vi "Get Min Max.vi"(10 "Axis":T1, 11 "Hailstone in":refnum<class "Hailstone.lvclass">) -> (3 "Limits":cluster{"Min":i64, "Max":i64})   [LabVIEW 2021, in "Hailstone.lvclass"]
uses:
  Hailstone.lvclass
  Axis.ctl
  Hailstone.lvclass/Hailstone.ctl
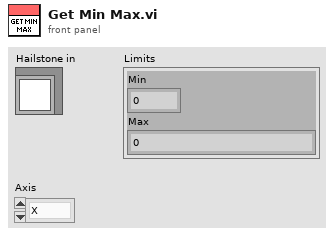
[diagram p1: front panel]
types:
  T1 = typedef "Hailstone.lvclass/Axis.ctl" = enum16{"X", "Y", "Z"}
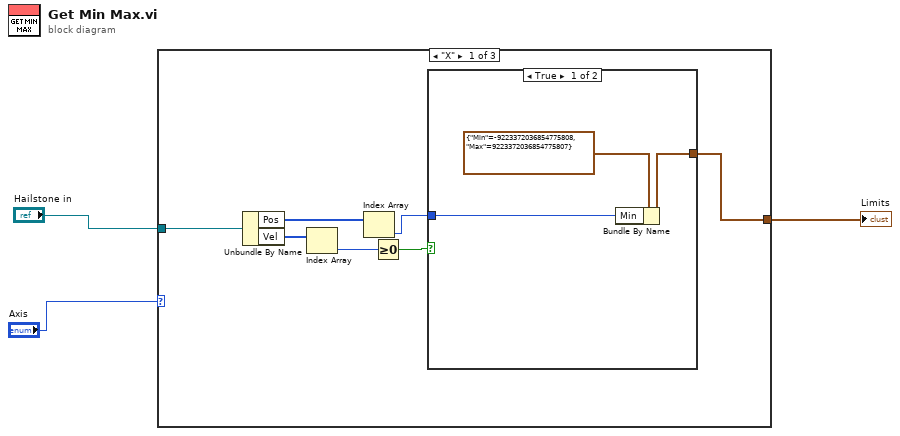
[diagram p0: block diagram]
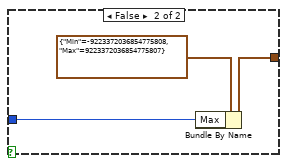
[diagram p2: hidden frame]
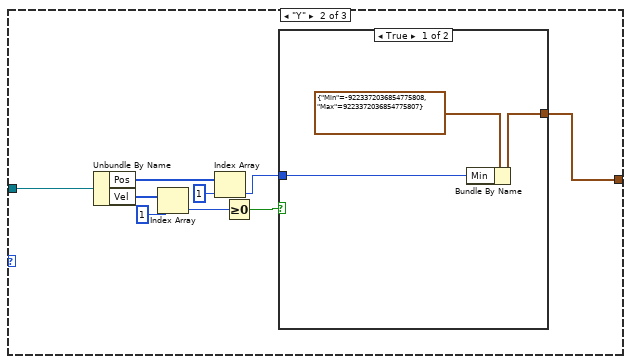
[diagram p3: hidden frame]
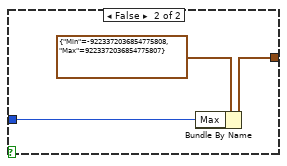
[diagram p4: hidden frame]
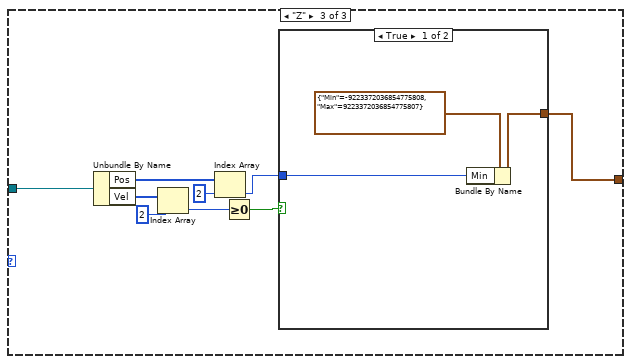
[diagram p5: hidden frame]
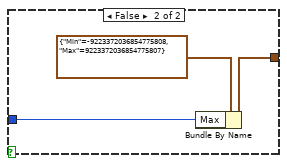
[diagram p6: hidden frame]
diagram:
  n1 = case shown="\"X\"" "Axis" {
    tunnel: "Hailstone in" -> [w10 w25 w40]
    tunnel: [w6 w21 w36] -> w2
    frame "X" {
      n2 = Unbundle By Name(w10) -> ("Pos"=w5:i64[], "Vel"=w9:i64[])
      n3 = Index Array(array=w9) -> (element=w8:i64)  [unwired: 1 in]
      n4 = Index Array(array=w5) -> (element=w4:i64)  [unwired: 1 in]
      n5 = Greater Or Equal To 0?(x=w8) -> (x >= 0?=w7:bool)
      n6 = case shown="True" w7 {
        tunnel: [w12 w15] -> w6
        tunnel: w4 -> [w11 w14]
        frame True {
          n7 = Bundle By Name(cluster=cluster{"Min":i64, "Max":i64} {"Min"=-9223372036854775808, "Max"=9223372036854775807} ("Limits"), "Min"=w11) -> (w12:cluster{"Min":i64, "Max":i64})
        }
        frame False {
          n8 = Bundle By Name(cluster=cluster{"Min":i64, "Max":i64} {"Min"=-9223372036854775808, "Max"=9223372036854775807} ("Limits"), "Max"=w14) -> (w15:cluster{"Min":i64, "Max":i64})
        }
      }
    }
    frame "Y" {
      n9 = Unbundle By Name(w25) -> ("Pos"=w20:i64[], "Vel"=w24:i64[])
      n10 = Index Array(array=w24, index=1) -> (element=w23:i64)
      n11 = Index Array(array=w20, index=1) -> (element=w19:i64)
      n12 = Greater Or Equal To 0?(x=w23) -> (x >= 0?=w22:bool)
      n13 = case shown="True" w22 {
        tunnel: [w27 w30] -> w21
        tunnel: w19 -> [w26 w29]
        frame True {
          n14 = Bundle By Name(cluster=cluster{"Min":i64, "Max":i64} {"Min"=-9223372036854775808, "Max"=9223372036854775807} ("Limits"), "Min"=w26) -> (w27:cluster{"Min":i64, "Max":i64})
        }
        frame False {
          n15 = Bundle By Name(cluster=cluster{"Min":i64, "Max":i64} {"Min"=-9223372036854775808, "Max"=9223372036854775807} ("Limits"), "Max"=w29) -> (w30:cluster{"Min":i64, "Max":i64})
        }
      }
    }
    frame "Z" {
      n16 = Unbundle By Name(w40) -> ("Pos"=w35:i64[], "Vel"=w39:i64[])
      n17 = Index Array(array=w39, index=2) -> (element=w38:i64)
      n18 = Index Array(array=w35, index=2) -> (element=w34:i64)
      n19 = Greater Or Equal To 0?(x=w38) -> (x >= 0?=w37:bool)
      n20 = case shown="True" w37 {
        tunnel: [w42 w45] -> w36
        tunnel: w34 -> [w41 w44]
        frame True {
          n21 = Bundle By Name(cluster=cluster{"Min":i64, "Max":i64} {"Min"=-9223372036854775808, "Max"=9223372036854775807} ("Limits"), "Min"=w41) -> (w42:cluster{"Min":i64, "Max":i64})
        }
        frame False {
          n22 = Bundle By Name(cluster=cluster{"Min":i64, "Max":i64} {"Min"=-9223372036854775808, "Max"=9223372036854775807} ("Limits"), "Max"=w44) -> (w45:cluster{"Min":i64, "Max":i64})
        }
      }
    }
  }
  "Limits" <- w2
